vi "FW_checkSubProcess.vi"(8 "error in":errorcluster, 9 "running? (F)":bool, 10 "Sub-process name":T1, 11 "Cluster":T2) -> (0 "error out":errorcluster, 2 "any process running":bool, 3 "Cluster out":T2)   [LabVIEW 2021, in "Framework_lib.lvlib"]
uses:
  QMH/Framework_lib.lvlib
  FW_producer_Cluster.ctl
  FW_producer_Data.ctl
  QMH/QMH_references_enum.ctl
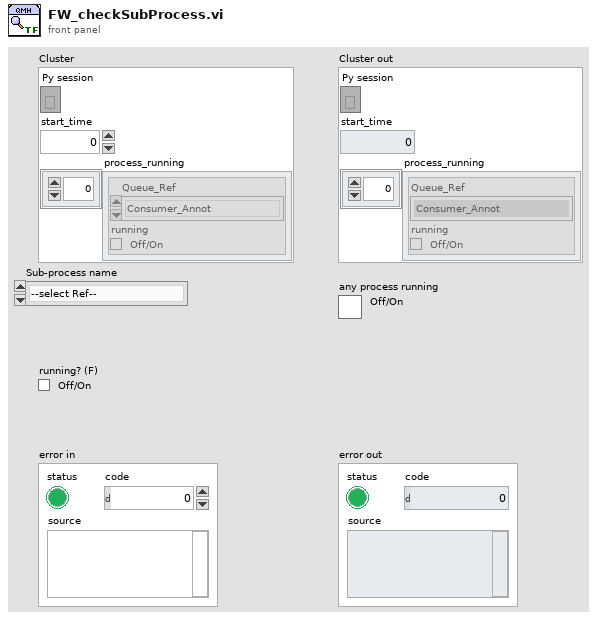
[diagram p1: front panel]
types:
  T1 = typedef "Framework_lib.lvlib/QMH_references_enum.ctl" = enum16{"--select Ref--", "Consumer_SUT", "Consumer_Annot", "Compute_Results"}
  T2 = typedef "Framework_lib.lvlib/FW_producer_Cluster.ctl" = cluster{"Py session":refnum<k35>, "start_time":u32, "process_running":T3[]}
  T3 = typedef "Framework_lib.lvlib/FW_producer_Data.ctl" = cluster{"Queue_Ref":T1, "running":bool}
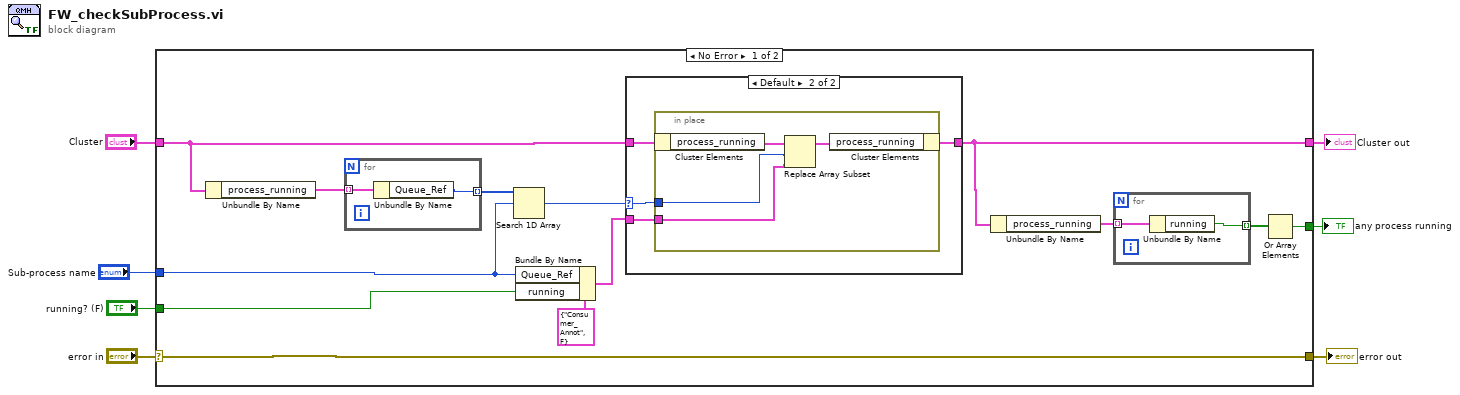
[diagram p0: block diagram]
diagram:
  n1 = case shown="No Error" "error in" {
    selector: "error in" -> [w8 w34]
    tunnel: "Cluster" -> [w20 _]
    tunnel: "running? (F)" -> [w15 _]
    tunnel: [w8 w34] -> w4
    tunnel: [w12 _] -> w3
    tunnel: [w10 _] -> w2
    tunnel: "Sub-process name" -> [w9 _]
    frame No Error {
      n2 = Unbundle By Name(w20) -> ("process_running"=w19:T3[])
      n3 = for {
        tunnel: w19 -> [w22] mode=indexing
        tunnel: [w21] -> w18 mode=indexing
        n4 = Unbundle By Name(w22) -> ("Queue_Ref"=w21:T1)
      }
      n5 = Search 1D Array(1D array=w18, element=w9) -> (index of element=w17:i32)  [unwired: 1 in]
      n6 = Bundle By Name(cluster=T3 {"Queue_Ref"=enum."Consumer_Annot", "running"=FALSE} ("process running"), "Queue_Ref"=w9, "running"=w15) -> (w14:T3)
      n7 = case shown="Default" w17 {
        selector: w17 -> [_ w26]
        tunnel: w20 -> [w23 w27]
        tunnel: w14 -> [_ w25]
        tunnel: [w23 w24] -> w12
        frame -1 {
        }
        frame Default {
          n8 = in-place {
            in-place-border: w26 -> [w30]
            in-place-border: w25 -> [w29]
            n9 = in-place-cluster #1(w27) -> ("process_running"=w31:T3[])
            n10 = Replace Array Subset(array=w31, new element=w29, index=w30) -> (w28:T3[])
            n11 = in-place-cluster #1("process_running"=w28) -> (w24:T2)
          }
        }
      }
      n12 = Unbundle By Name(w12) -> ("process_running"=w13:T3[])
      n13 = for {
        tunnel: w13 -> [w33] mode=indexing
        tunnel: [w32] -> w11 mode=indexing
        n14 = Unbundle By Name(w33) -> ("running"=w32:bool)
      }
      n15 = Or Array Elements(Boolean array=w11) -> (logical OR=w10:bool)
    }
    frame Error {
    }
  }
  "any process running" <- w2
  "error out" <- w4
  "Cluster out" <- w3
